vi "Samle SG05p.vi"() -> ()   [LabVIEW 2009]
uses:
  SubVI/Settings.ctl
  Extra/MGI Change Detector (T).vi
panel:
  in  "External\nPrescaler":u16=4 min=1 max=32
  in  "Internal\nPrescaler":u16=6 min=1 max=32
  in  "Trigger\nInhibit (ms)":dbl=0.2 min=0.0001 max=50000.0 step=0.1 format="%.4f"
  in  "Settings":T1={"T Delay (µs)"=0.0, "T Set Back"=0.0, "T Triggers"=0, "T Active"=TRUE, "T Polarity"=TRUE, "T Term"=TRUE, "T Drive"=FALSE, "A Delay (µs)"=0.0, "A Set Back"=0.0, "A Triggers"=0, "A Active"=TRUE, "A Polarity"=TRUE, "A Term"=TRUE, "A Drive"=FALSE, "B Delay (µs)"=0.0, "B Set Back"=0.0, "B Triggers"=0, "B Active"=TRUE, "B Polarity"=TRUE, "B Term"=TRUE, "B Drive"=FALSE, "Gate A*B"=FALSE, "Output\nLevel"=1, "Trigger\nTerminate"=TRUE, "Clock\nEnable"=TRUE, "Internal\nClock (µs)"=0.0125, "Trigger\nLevel"=0.2, "Stop\nTrigger"=1, "Ocillator\nDivide By"=6, "Clock Source"=3, "Gate Divider"=1, "Positive\nGate"=FALSE, "Trigger\nSource"=FALSE, "Internal\nArming"=FALSE, "Software\nTrigger"=FALSE, "Trigger\nSlope"=TRUE, "Stop on\nPreset"=FALSE, "Trigger\nOperation"=TRUE, "Trigger\nEnable"=TRUE} {"B Set Back" min=0.0 format="%.3f"; "A Set Back" min=0.0 format="%.3f"; "T Set Back" min=0.0 format="%.3f"; "Clock Source" items=["Internal Oscillator"=1, "External Trigger"=2, "Trigger & Oscillator"=3, "Master Slave Bus"=4]; "Trigger\nLevel" min=0.0 format="%.3f"; "Output\nLevel" items=["TTL"=1, "NIM"=2, "ECL"=3]; "Internal\nClock (µs)" min=0.0 format="%.4f"; "B Delay (µs)" min=0.0 format="%.3f"; "A Delay (µs)" min=0.0 format="%.3f"; "T Delay (µs)" min=0.0 format="%.3f"}
  in  "Pulse Width":u32=2 min=2 max=255
  in  "Clock Source":u32(ring)=3 items=["Internal Oscillator"=1, "External Trigger"=2, "Trigger & Oscillator"=3, "Master Slave Bus"=4]
  in  "Internal\nArming":bool
  in  "B HighDrive":bool
  in  "B Terminaton":bool=TRUE
  in  "B Polarity":bool=TRUE
  in  "B activity":bool=TRUE
  in  "B Extra Delay (ms)":dbl min=0.0 max=100000000.0 format="%.5f"
  in  "A HighDrive":bool
  in  "A Terminaton":bool=TRUE
  in  "A Polarity":bool=TRUE
  in  "A activity":bool=TRUE
  in  "A Extra Delay (ms)":dbl min=0.0 max=100000000.0 format="%.5f"
  in  "T HighDrive":bool
  in  "T Terminaton":bool=TRUE
  in  "T Polarity":bool=TRUE
  in  "T Extra Delay (ms)":dbl min=0.0 max=100000000.0 format="%.5f"
  in  "T activity":bool=TRUE
  in  "Operation":bool=TRUE
  in  "Stop On Preset":bool
  in  "Software Trigger":bool
  in  "Positive Gate":bool
  in  "Gate AB":bool
  in  "Clock":bool=TRUE
  in  "Output":bool=TRUE
  in  "Slope":bool=TRUE
  in  "Input\nImpedance":bool=TRUE
  in  "Trigger Source":bool
  in  "Internal\nRate (µs)":dbl=0.0125 min=0.0125 max=50.0 format="%.4f"
  in  "Output Level":u32(ring)=1 items=["TTL"=1, "NIM"=2, "ECL"=3]
  in  "Gate Divider":u32=1 min=1 max=1000000
  in  "Preset":u32=1 max=10000000
  in  "External Trigger\nLevel (V)":dbl=0.2 min=-2.5 max=2.5 format="%.2f"
  in  "Activate":bool
  in  "Stop":bool
  out "DG Product":i32(ring)=39 items=["SRS_DG135"=1, "BME_DP01"=2, "BME_G02V3"=3, "BME_SG02V4"=4, "BME_G04"=5, "BME_G02V1"=6, "BME_G02V2"=7, "BME_SG02V1"=8, "BME_SG02V2"=9, "BME_SG02V3"=10, "BME_G03V1"=11, "BME_G03V2"=12, "BME_SG02V5"=13, "BME_G03V3"=14, "BME_G03V4"=15, "BME_SG02V6"=16, "BME_G03V5"=17, "BME_G05V1"=18, "BME_G05V2"=19, "BME_G05V3"=20, "BME_SG02V7"=21, "BME_SG02P1"=31, "BME_G03P1"=32, "BME_G05P1"=33, "BME_SG02P2"=34, "BME_G03P2"=35, "BME_SG02P3"=36, "BME_SG05P1"=37, "BME_G05P2"=38, "BME_SG05P2"=39, "BME_G05P3"=40, "BME_SG02P4"=41]
  out "Slot Number":i32=4
  out "Master":bool=TRUE
  out "DG_Number":i32
  # "Delay Generator Control"
  # "BME Card Information"
  # "Output Channel Settings"
  # "State"
  # "Polarity"
  # "Delay (µs)"
  # "50 ohm Output"
  # "25 ohm Output"
  # "T"
  # "A"
  # "B"
  # "Output Settings"
  # "Clock Settings"
  # "Trigger Settings"
  # "NOTICE -- YOU MUST LEAVE THIS NOTICE IN PLACE.  PER THE TERMS OF THE LICENSE BELOW, YOU MAY SUBLICENSE THIS SOFTWARE \nIN ANY WAY THAT DOES NOT CONFLICT WITH THIS LICENSE.\n\n### BSD License (http://www.opensource.org/licenses/bsd-license.php) Begin ###\n \nCopyright (c) 2011, Applied Energetics, http://www.appliedenergetics.com,\n                               Richard Schwerdtfeger, <rschwerdtfeger@appliedenergetics.com>\n\nAll rights reserved.\n\nRedistribution and use in source and binary forms, with or without modification, are permitted provided that the \nfollowing conditions are met:\n\n    * Redistributions of source code must retain the above copyright notice, this list of conditions and the following disclaimer.\n    * Redistributions in binary form must reproduce the above copyright notice, this list of conditions and the following disclaimer \n       in the documentation and/or other materials provided with the distribution.\n    * Neither the name of Richard Schwerdtfeger, Applied Energetics, Inc., nor the names of its contributors may be used to \n       endorse or promote products derived from this software without specific prior written permission.\n\nTHIS SOFTWARE IS PROVIDED BY THE COPYRIGHT HOLDERS AND CONTRIBUTORS \"AS IS\" AND ANY EXPRESS OR IMPLIED WARRANTIES, \nINCLUDING, BUT NOT LIMITED TO, THE IMPLIED WARRANTIES OF MERCHANTABILITY AND FITNESS FOR A PARTICULAR PURPOSE ARE \nDISCLAIMED. IN NO EVENT SHALL THE COPYRIGHT OWNER OR CONTRIBUTORS BE LIABLE FOR ANY DIRECT, INDIRECT, INCIDENTAL,\n SPECIAL, EXEMPLARY, OR CONSEQUENTIAL DAMAGES (INCLUDING, BUT NOT LIMITED TO, PROCUREMENT OF SUBSTITUTE GOODS OR \nSERVICES; LOSS OF USE, DATA, OR PROFITS; OR BUSINESS INTERRUPTION) HOWEVER CAUSED AND ON ANY THEORY OF LIABILITY, \nWHETHER IN CONTRACT, STRICT LIABILITY, OR TORT (INCLUDING NEGLIGENCE OR OTHERWISE) ARISING IN ANY WAY OUT OF THE USE \nOF THIS SOFTWARE, EVEN IF ADVISED OF THE POSSIBILITY OF SUCH DAMAGE.\n\n### BSD License End ###"
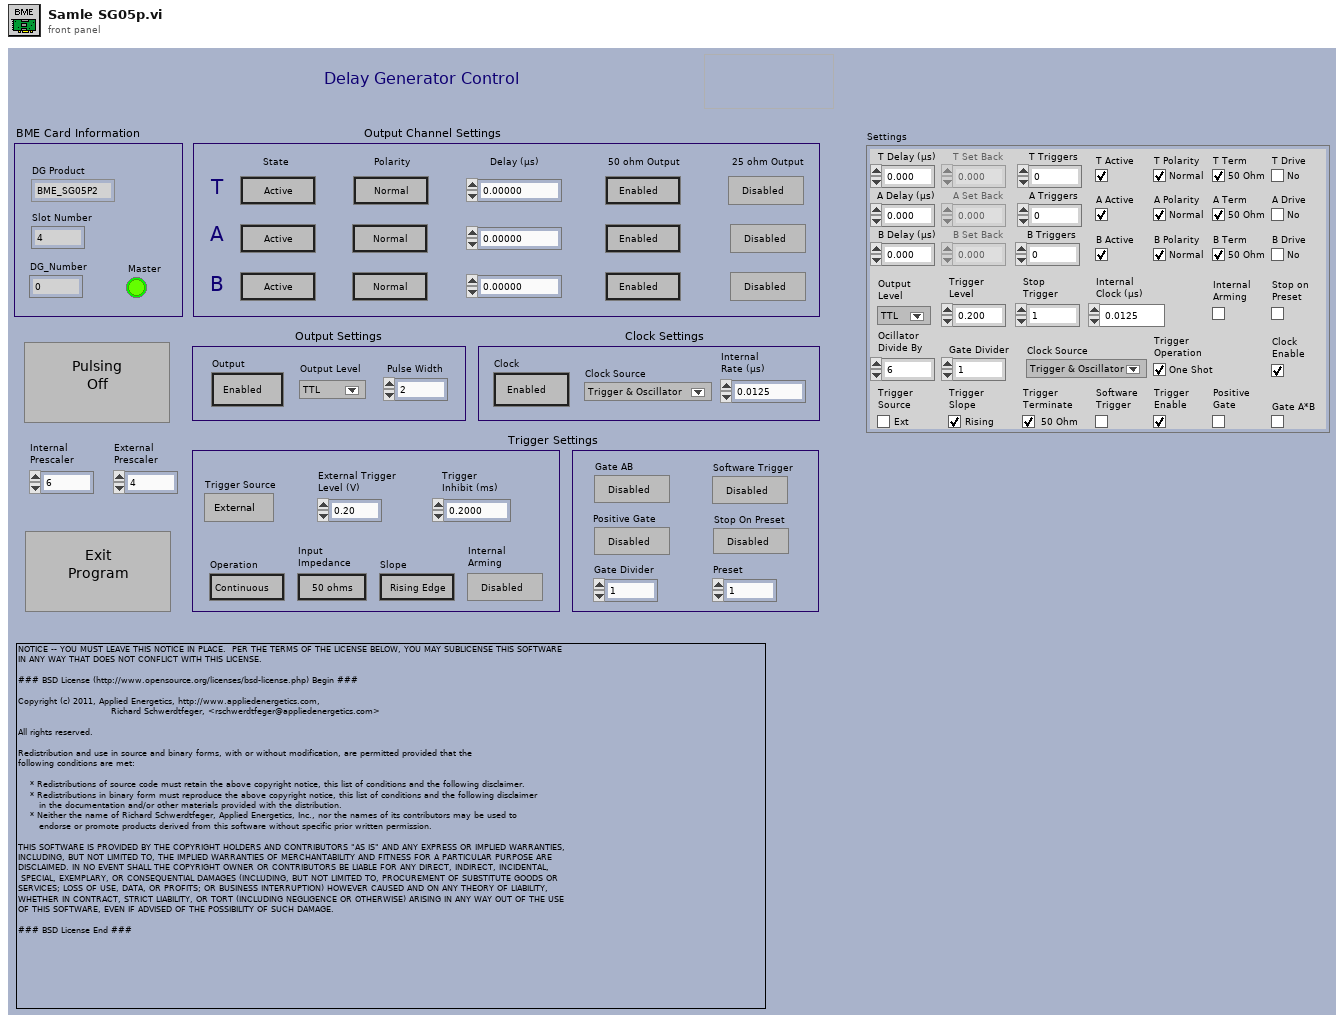
[diagram p1: front panel]
types:
  T1 = typedef "Settings.ctl" = cluster{"T Delay (µs)":dbl, "T Set Back":dbl, "T Triggers":u16, "T Active":bool, "T Polarity":bool, "T Term":bool, "T Drive":bool, "A Delay (µs)":dbl, "A Set Back":dbl, "A Triggers":u16, "A Active":bool, "A Polarity":bool, "A Term":bool, "A Drive":bool, "B Delay (µs)":dbl, "B Set Back":dbl, "B Triggers":u16, "B Active":bool, "B Polarity":bool, "B Term":bool, "B Drive":bool, "Gate A*B":bool, "Output\nLevel":u32, "Trigger\nTerminate":bool, "Clock\nEnable":bool, "Internal\nClock (µs)":dbl, "Trigger\nLevel":dbl, "Stop\nTrigger":u32, "Ocillator\nDivide By":u16, "Clock Source":u32, "Gate Divider":u32, "Positive\nGate":bool, "Trigger\nSource":bool, "Internal\nArming":bool, "Software\nTrigger":bool, "Trigger\nSlope":bool, "Stop on\nPreset":bool, "Trigger\nOperation":bool, "Trigger\nEnable":bool}
  T2 = cluster{"DG Product":i32, "Slot Number":i32, "Master":bool, "DG Number":i32}[]
  T3 = cluster{"DG Product":i32, "Slot Number":i32, "Master":bool, "DG Number":i32}
  T4 = enum8{"Enabled", "Disabled", "Disabled and Grayed Out"}
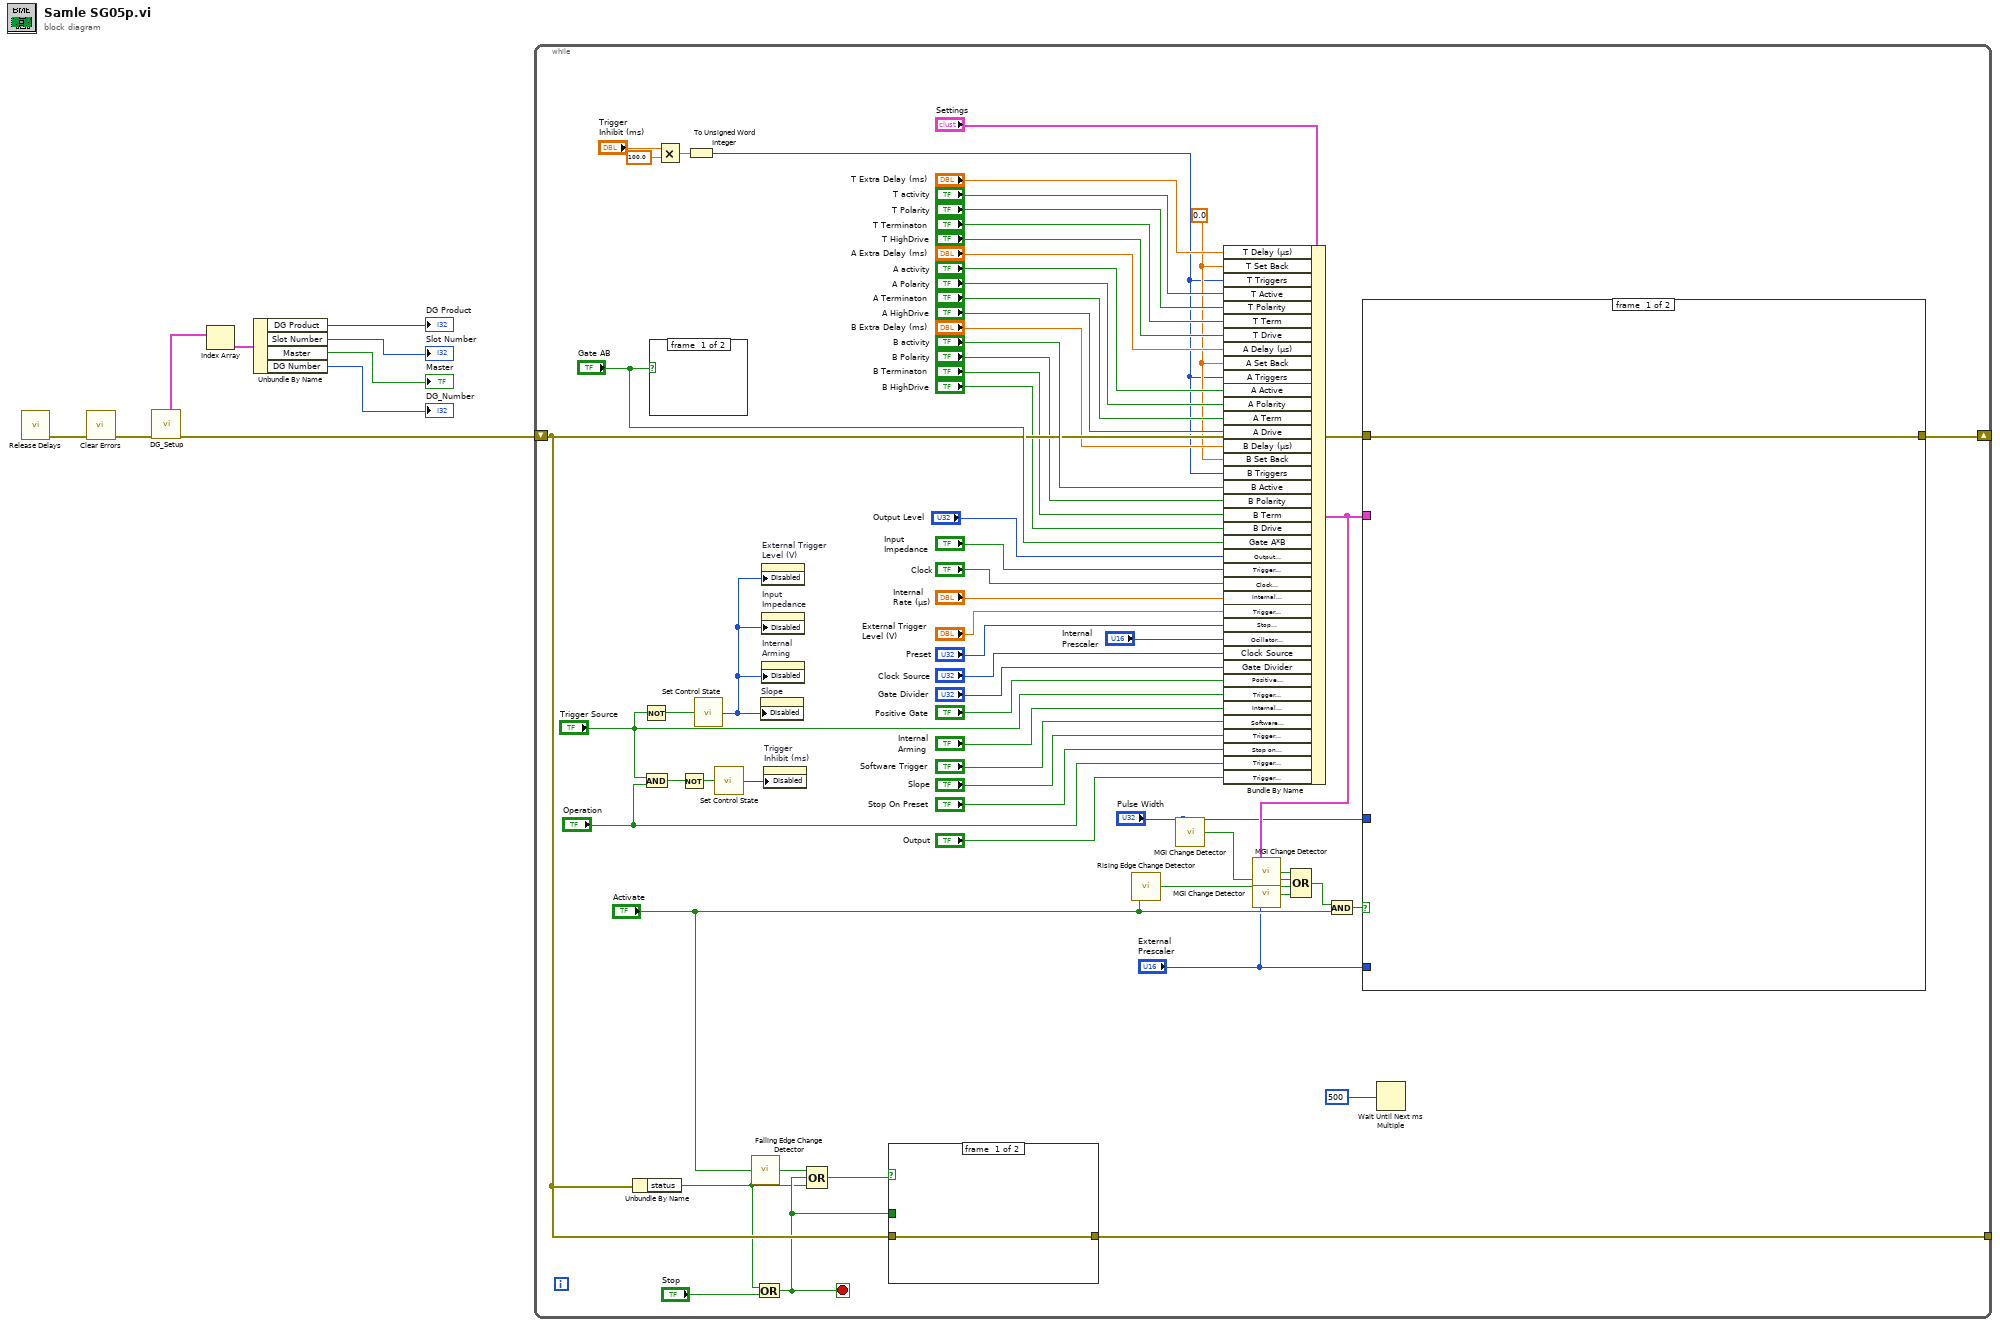
[diagram p0: block diagram]
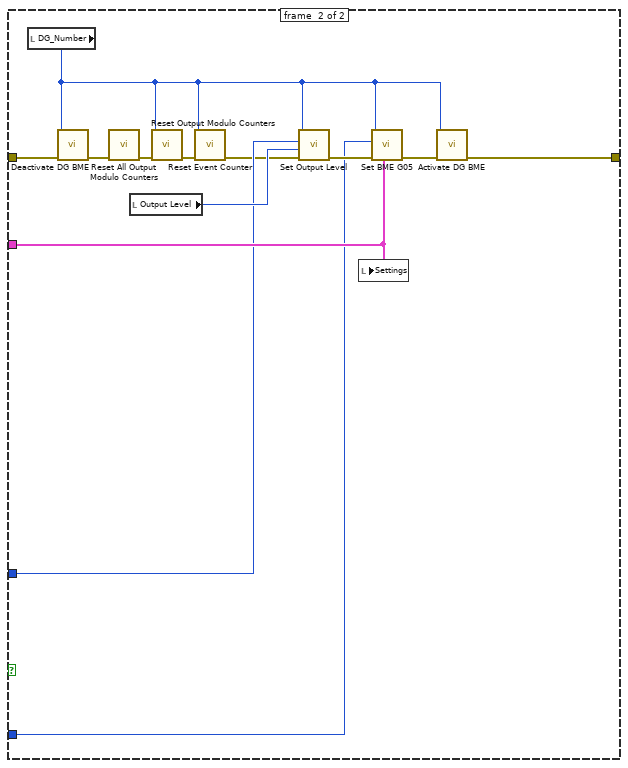
[diagram p2: hidden frame]
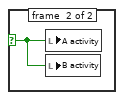
[diagram p3: hidden frame]
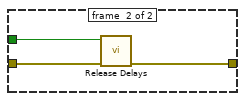
[diagram p4: hidden frame]
diagram:
  n1 = call "Release Delays.vi"() -> ("error out"=w3:errorcluster)  [unwired: 2 in, 9 out]
  n2 = call <vilib>:"Clear Errors.vi"("error in (no error)"=w3) -> ("error out"=w2:errorcluster)  [unwired: 6 out]
  n3 = call "DG_Setup.vi"("error in (no error)"=w2) -> ("error out"=w4:errorcluster, "Generator Info"=w1:T2)  [unwired: 2 in, 7 out]
  n4 = Index Array(array=w1) -> (element=w5:T3)  [unwired: 1 in]
  n5 = Unbundle By Name(w5) -> ("DG Product"=→"DG Product":i32, "Slot Number"=→"Slot Number":i32, "Master"=→"Master":bool, "DG Number"=→"DG_Number":i32)
  n6 = while {
    shift-right: [w68] -> _
    shift-left: w4 -> [w64]
    tunnel: [w14] -> _
    stop <- w63 stop-if-true
    w50 = 0.0 ("T0 Set Back")
    n7 = Unbundle By Name(w64) -> ("status"=w61:bool)
    n8 = Not(x="Trigger Source") -> (.not. x?=w19:bool)
    n9 = And(x="Trigger Source", y="Operation") -> (x .and. y?=w24:bool)
    n10 = case shown="True" "Gate AB" {
      selector: "Gate AB" -> [_ w87]
      frame #0 {
      }
      frame #1 {
        n11 = local write "A activity"(w87) -> ()
        n12 = local write "B activity"(w87) -> ()
      }
    }
    n13 = Multiply(x="Trigger\nInhibit (ms)", y=100.0) -> (x*y=w22:dbl)
    n14 = Not(x=w24) -> (.not. x?=w21:bool)
    n15 = To Unsigned Word Integer(number=w22) -> (unsigned 16bit integer=w15:u16)
    n16 = call "Set Control State.vi"("Enable"=w19) -> ("State"=w18:T4)  [unwired: 4 out]
    n17 = call "Set Control State.vi"("Enable"=w21) -> ("State"=w20:T4)  [unwired: 4 out]
    n18 = call "Falling Edge Change Detector.vi"("Input Value"="Activate") -> ("Falling Edge?"=w60:bool)  [unwired: 4 out]
    n19 = Or(x=w61, y="Stop") -> (x .or. y?=w63:bool)
    n20 = property on="Slope" class="Bool (strict)"("Disabled"=w18) -> ()  [unwired: 2 in, 2 out]
    n21 = property on="External Trigger\nLevel (V)" class="DigNum (strict)"("Disabled"=w18) -> ()  [unwired: 2 in, 2 out]
    n22 = property on="Input\nImpedance" class="Bool (strict)"("Disabled"=w18) -> ()  [unwired: 2 in, 2 out]
    n23 = property on="Internal\nArming" class="Bool (strict)"("Disabled"=w18) -> ()  [unwired: 2 in, 2 out]
    n24 = property on="Trigger\nInhibit (ms)" class="DigNum (strict)"("Disabled"=w20) -> ()  [unwired: 2 in, 2 out]
    n25 = Compound Arithmetic op=OR(w60, w63, w61) -> (w71:bool)
    n26 = case shown="True" w71 {
      tunnel: w63 -> [_ w90]
      tunnel: w64 -> [w88 w91]
      tunnel: [w88 w89] -> w14
      frame #0 {
      }
      frame #1 {
        n27 = call "Release Delays.vi"("error in (no error)"=w91, "Release"=w90) -> ("error out"=w89:errorcluster)  [unwired: 9 out]
      }
    }
    n28 = call "Rising Edge Change Detector.vi"("Input Value"="Activate") -> ("Rising Edge?"=w25:bool)  [unwired: 4 out]
    n29 = call-poly "MGI Change Detector.vi"("Value"="Pulse Width") -> ("Changed?"=w12:bool)
    n30 = Bundle By Name(cluster="Settings", "T Delay (µs)"="T Extra Delay (ms)", "T Set Back"=w50, "T Triggers"=w15, "T Active"="T activity", "T Polarity"="T Polarity", "T Term"="T Terminaton", "T Drive"="T HighDrive", "A Delay (µs)"="A Extra Delay (ms)", "A Set Back"=w50, "A Triggers"=w15, "A Active"="A activity", "A Polarity"="A Polarity", "A Term"="A Terminaton", "A Drive"="A HighDrive", "B Delay (µs)"="B Extra Delay (ms)", "B Set Back"=w50, "B Triggers"=w15, "B Active"="B activity", "B Polarity"="B Polarity", "B Term"="B Terminaton", "B Drive"="B HighDrive", "Gate A*B"="Gate AB", "Output\nLevel"="Output Level", "Trigger\nTerminate"="Input\nImpedance", "Clock\nEnable"="Clock", "Internal\nClock (µs)"="Internal\nRate (µs)", "Trigger\nLevel"="External Trigger\nLevel (V)", "Stop\nTrigger"="Preset", "Ocillator\nDivide By"="Internal\nPrescaler", "Clock Source"="Clock Source", "Gate Divider"="Gate Divider", "Positive\nGate"="Positive Gate", "Trigger\nSource"="Trigger Source", "Internal\nArming"="Internal\nArming", "Software\nTrigger"="Software Trigger", "Trigger\nSlope"="Slope", "Stop on\nPreset"="Stop On Preset", "Trigger\nOperation"="Operation", "Trigger\nEnable"="Output") -> (w28:T1)
    n31 = call-poly "MGI Change Detector.vi"("Value"=w28) -> ("Changed?"=w27:bool)
    n32 = call-poly "MGI Change Detector.vi"("Value"="External\nPrescaler") -> ("Changed?"=w11:bool)
    n33 = Compound Arithmetic op=OR(w27, w12, w25, w11) -> (w29:bool)
    n34 = And(x=w29, y="Activate") -> (x .and. y?=w30:bool)
    n35 = case shown="True" w30 {
      tunnel: [w73 w76] -> w68
      tunnel: w64 -> [w73 w86]
      tunnel: w28 -> [_ w85]
      tunnel: "Pulse Width" -> [_ w83]
      tunnel: "External\nPrescaler" -> [_ w74]
      frame #0 {
      }
      frame #1 {
        n36 = local read "DG_Number"() -> (w75:i32)
        n37 = call "Deactivate DG BME.vi"("error in (no error)"=w86, "DG Number"=w75) -> ("error out"=w81:errorcluster)  [unwired: 9 out]
        n38 = call "Reset All Output Modulo Counters.vi"("error in (no error)"=w81) -> ("error out"=w80:errorcluster)  [unwired: 10 out]
        n39 = local read "Output Level"() -> (w84:u32)
        n40 = call "Reset Output Modulo Counters.vi"("error in (no error)"=w80, "DG Number"=w75) -> ("error out"=w79:errorcluster)  [unwired: 9 out]
        n41 = call "Reset Event Counter.vi"("error in (no error)"=w79, "DG Number"=w75) -> ("error out"=w78:errorcluster)  [unwired: 9 out]
        n42 = call "Set Output Level.vi"("error in (no error)"=w78, "Output Level"=w84, "Pulse Width"=w83, "DG Number"=w75) -> ("error out"=w82:errorcluster)  [unwired: 7 out]
        n43 = local write "Settings"(w85) -> ()
        n44 = call "Set BME G05.vi"("Settings"=w85, "error in (no error)"=w82, "External Prescaler"=w74, "DG Number"=w75) -> ("error out"=w77:errorcluster)  [unwired: 7 out]
        n45 = call "Activate DG BME.vi"("error in (no error)"=w77, "DG Number"=w75) -> ("error out"=w76:errorcluster)  [unwired: 9 out]
      }
    }
    n46 = Wait Until Next ms Multiple(millisecond multiple=u32 500) -> ()  [unwired: 1 out]
  }
